vi "allocate image memory.vi"(0 "Thorcam in":refnum<class "Thorcam.lvclass">, 1 "runtime.handles.camera handle":u32, 5 "error in (no error)":errorcluster) -> (10 "ColorMode":i32, 11 "Width":i32, 12 "Bits/Pixel":i32, 13 "Height":i32, 14 "Thorcam out":refnum<class "Thorcam.lvclass">, 15 "Camera Handle Out":u32, 17 "Memory ID Out":i32, 18 "Image Memory Out":u8[](array[numeric]), 19 "error out":errorcluster)   [LabVIEW 2012, in "Thorcam.lvclass"]
uses:
  Thorcam.lvclass
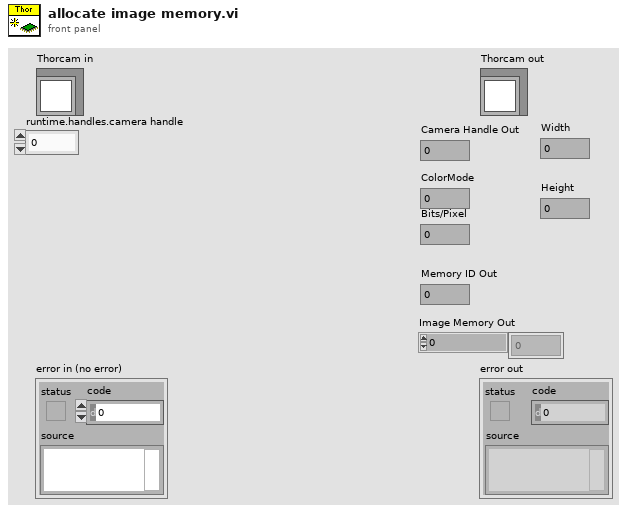
[diagram p1: front panel]
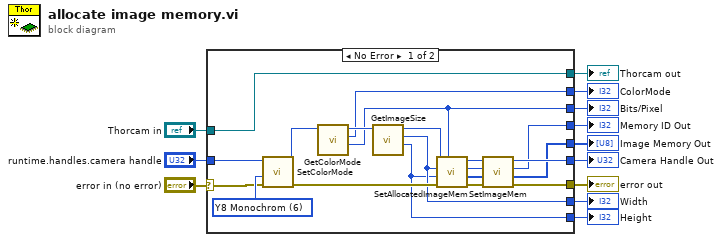
[diagram p0: block diagram]
diagram:
  n1 = case shown="No Error" "error in (no error)" {
    selector: "error in (no error)" -> [w29 w34]
    tunnel: [w24 w34] -> w11
    tunnel: [w16 w33] -> w10
    tunnel: "Thorcam in" -> [w16 w33]
    tunnel: "runtime.handles.camera handle" -> [w28 _]
    tunnel: [w22 _] -> w7
    tunnel: [w19 _] -> w6
    tunnel: [w18 _] -> w5
    tunnel: [w15 _] -> w4
    tunnel: [w14 _] -> w3
    tunnel: [w17 _] -> w2
    tunnel: [w13 _] -> w1
    frame No Error {
      w30 = 6 items=["RGB 32"=0, "RGB 24"=1, "Y8 Monochrom"=6] ("Mode")
      n2 = call <instrlib>:"SetColorMode.vi"("error in"=w29, "Mode"=w30, "Camera Handle In"=w28) -> ("error out"=w27:errorcluster, "Camera Handle Out"=w31:u32)  [unwired: 7 in]
      n3 = call <instrlib>:"GetColorMode.vi"("Camera Handle In"=w31) -> ("Bits/Pixel"=w13:i32, "ColorMode"=w17:i32, "Camera Handle Out"=w32:u32)  [unwired: 8 in]
      n4 = call <instrlib>:"GetImageSize.vi"("Camera Handle In"=w32) -> ("Height"=w14:i32, "Width"=w15:i32, "Camera Handle Out"=w26:u32)  [unwired: 8 in]
      n5 = call <instrlib>:"SetAllocatedImageMem.vi"("BitsPixel"=w13, "error in"=w27, "Height"=w14, "Width"=w15, "Camera Handle In"=w26) -> ("error out"=w25:errorcluster, "Image Memory Out"=w20:u8[], "Memory ID Out"=w21:i32, "Camera Handle Out"=w23:u32)  [unwired: 2 in, 1 out]
      n6 = call <instrlib>:"SetImageMem.vi"("error in"=w25, "Image Memory In"=w20, "Memory ID In"=w21, "Camera Handle In"=w23) -> ("error out"=w24:errorcluster, "Image Memory Out"=w18:u8[], "Memory ID Out"=w19:i32, "Camera Handle Out"=w22:u32)  [unwired: 4 in]
    }
    frame Error {
    }
  }
  "error out" <- w11
  "Thorcam out" <- w10
  "Camera Handle Out" <- w7
  "ColorMode" <- w2
  "Bits/Pixel" <- w1
  "Width" <- w4
  "Height" <- w3
  "Memory ID Out" <- w6
  "Image Memory Out" <- w5
